vi "UpdateParams.vi"(8 "error in (no error)":errorcluster, 10 "Parameters":variant, 11 "ExpID":string) -> (0 "error out":errorcluster)   [LabVIEW 2017]
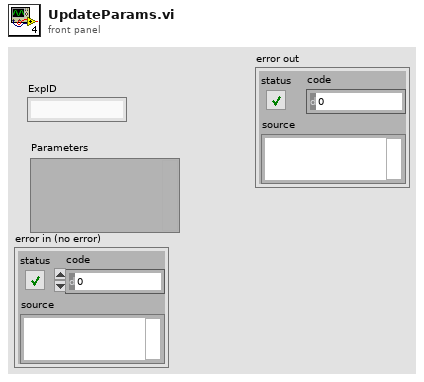
[diagram p1: front panel]
types:
  T1 = cluster{"MatlabType":u16, "Data":variant, "name":string}[]
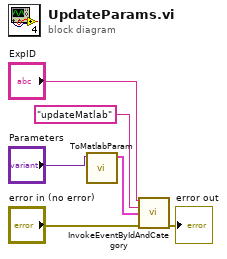
[diagram p0: block diagram]
diagram:
  n1 = call "ToMatlabParam.vi"("Value"="Parameters") -> ("Parameters"=w1:T1)  [unwired: 10 in]
  n2 = call "InvokeEventByIdAndCategory.vi"("ID"="ExpID", "eventName"="updateMatlab" ("name"), "Data"=w1, "error in (no error)"="error in (no error)") -> ("error out"=→"error out":errorcluster)  [unwired: 11 in]
